vi "Init.vi"(8 "error in (no error)":errorcluster, 11 "uPlugin_Handler in":refnum<class "uPlugin_Handler.lvclass">) -> (0 "error out":errorcluster)   [LabVIEW 2021, in "uPlug.lvlib" / "uPlugin_Handler.lvclass"]
doc: "Use to load a plugin-handler child class into memory."
uses:
  uPlugin_Handler.lvclass
  TypeDef_FGV Actions.ctl
  uPlugin_Handler.lvclass/uPlugin_Handler.ctl
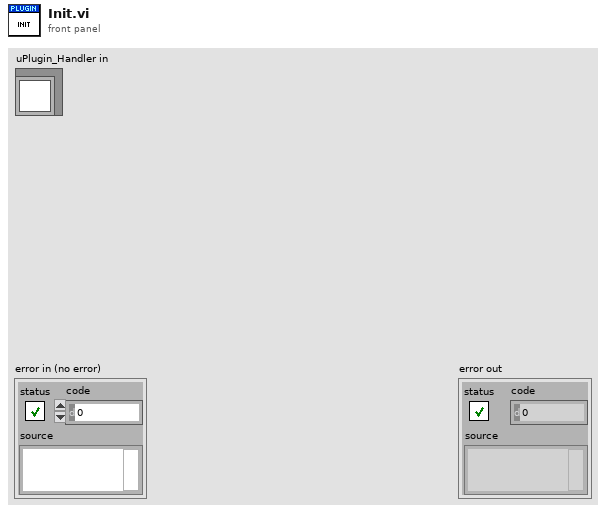
[diagram p1: front panel]
types:
  T1 = typedef "uPlug.lvlib/uPlugin_Handler.lvclass/TypeDef_FGV Actions.ctl" = enum16{"Init", "Load"}
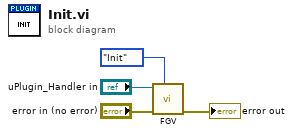
[diagram p0: block diagram]
diagram:
  n1 = call "FGV.vi"("Action"=TypeDef_FGV_Actions."Init", "error in (no error)"="error in (no error)", "iPlugin_Loader In"="uPlugin_Handler in") -> ("error out"=→"error out":errorcluster)  [unwired: 7 in, 1 out]
